vi "Setup Prepend to Log.vi"() -> (2 "Logger 2":string, 3 "Logger 1":string)   [LabVIEW 2023]
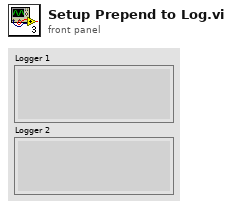
[diagram p1: front panel]
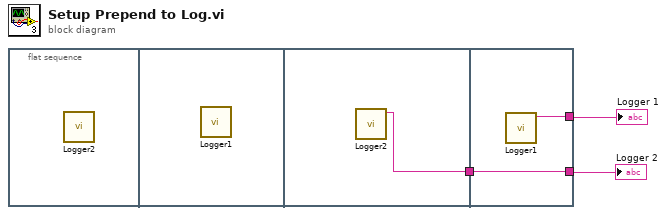
[diagram p0: block diagram]
diagram:
  n1 = flat-sequence {
    tunnel: [w4] -> w3
    tunnel: [w6] -> w1
    tunnel: [w5] -> w2
    tunnel: w3 -> [w5]
    frame #0 {
      n2 = call "Logger2.vi"() -> ()  [unwired: 11 in, 1 out]
    }
    frame #1 {
      n3 = call "Logger1.vi"() -> ()  [unwired: 11 in, 1 out]
    }
    frame #2 {
      n4 = call "Logger2.vi"() -> ("Log out"=w4:string)  [unwired: 11 in]
    }
    frame #3 {
      n5 = call "Logger1.vi"() -> ("Log out"=w6:string)  [unwired: 11 in]
    }
  }
  "Logger 2" <- w2
  "Logger 1" <- w1
